vi "readYearMonth.vi"(8 "error in (no error)":errorcluster, 11 "MonthDisplay in":refnum<class "DateUserInterface.lvclass">) -> (0 "error out":errorcluster, 2 "WhichMonth.lvclass":refnum<class "WhichMonth.lvclass">, 3 "MonthDisplay out":refnum<class "DateUserInterface.lvclass">)   [LabVIEW 2018, in "DateUserInterface.lvclass"]
uses:
  DateUserInterface.lvclass
  WhichMonth/WhichMonth.lvclass
  DateUserInterface.lvclass/DateUserInterface.ctl
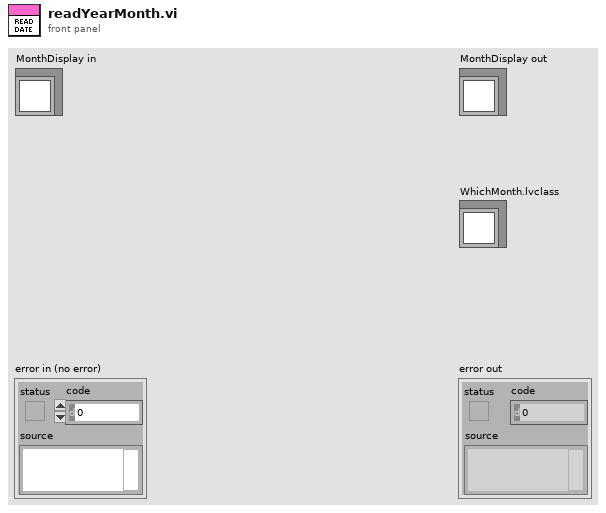
[diagram p1: front panel]
types:
  T1 = typedef "MonthDisplay.lvclass/month.ctl" = enum16{"January", "February", "March", "April", "May", "June", "July", "August", "September", "October", "November", "December"}
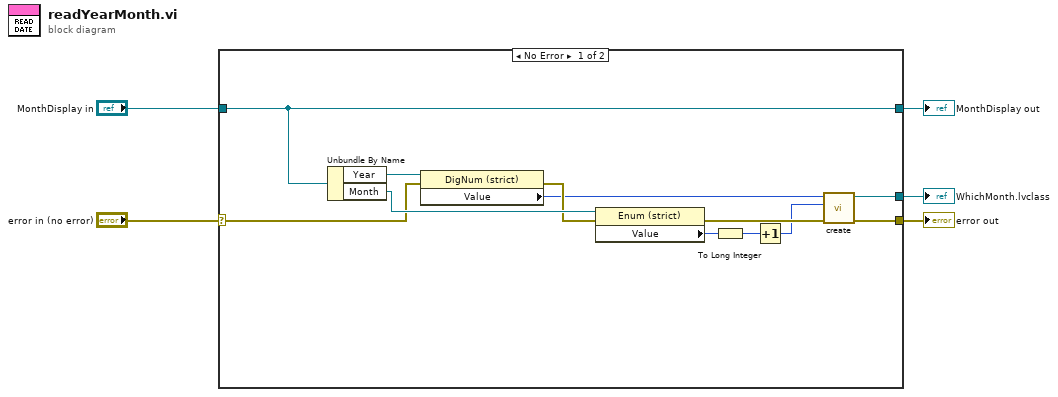
[diagram p0: block diagram]
diagram:
  n1 = case shown="No Error" "error in (no error)" {
    selector: "error in (no error)" -> [w14 w19]
    tunnel: [w10 w19] -> w4
    tunnel: [w17 w18] -> w2
    tunnel: "MonthDisplay in" -> [w17 w18]
    tunnel: [w11 _] -> w1
    frame No Error {
      n2 = Unbundle By Name(w17) -> ("Year"=w16:refnum<vi>, "Month"=w15:refnum<vi>)
      n3 = property class="DigNum (strict)"(reference=w16, error in=w14) -> (error out=w13:errorcluster, "Value"=w12:i32)  [unwired: 1 out]
      n4 = property class="Enum (strict)"(reference=w15, error in=w13) -> (error out=w9:errorcluster, "Value"=w8:T1)  [unwired: 1 out]
      n5 = To Long Integer(number=w8) -> (32bit integer=w7:i32)
      n6 = Increment(x=w7) -> (x+1=w6:i32)
      n7 = call "create.vi"("error in (no error)"=w9, "Month"=w6, "Year"=w12) -> ("error out"=w10:errorcluster, "WhichMonth out"=w11:refnum<class "WhichMonth.lvclass">)  [unwired: 7 in]
    }
    frame Error {
    }
  }
  "error out" <- w4
  "MonthDisplay out" <- w2
  "WhichMonth.lvclass" <- w1
